vi "Test Integration.vi"(1 "Integrated Signal":dynamicdata(graph), 2 "Signal In":dynamicdata(graph)) -> (0 "Equal":bool)   [LabVIEW 2010]
uses:
  Instance           1 24Saved   Test Integration .vi
  Instance           2 24Saved   Test Integration .vi
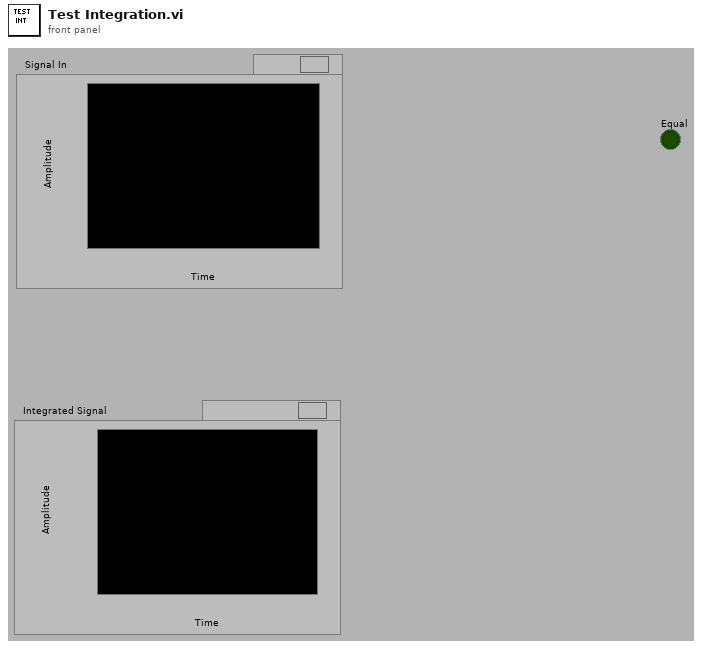
[diagram p1: front panel]
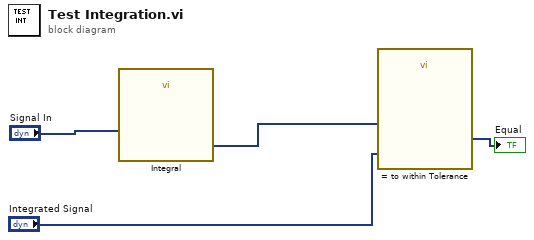
[diagram p0: block diagram]
diagram:
  n1 = call "Integral"("Signals"="Signal In") -> ("Result"=w3:dynamicdata)  [unwired: 1 in, 5 out]
  n2 = call "= to within Tolerance"("Operand 2"="Integrated Signal", "Operand 1"=w3) -> ("Result"=→"Equal":dynamicdata)  [unwired: 1 in, 8 out]
